vi "CameraQueryProperties.vi"(8 "error in (no error)":errorcluster, 11 "AndorSDK2 in":refnum<class "Andor3.lvclass">) -> (0 "error out":errorcluster, 1 "sensor_height":u16, 2 "sensor_width":u16, 3 "AndorSDK2 out":refnum<class "Andor3.lvclass">, 4 "cam_params":cluster{"String":string, "value":variant}[](array[cluster]) caption="params")   [LabVIEW 2010, in "Andor3.lvclass"]
uses:
  Andor3.lvclass
  Andor3.lvclass/Andor3.ctl
  <userlib>/atcoreA/atcoreA.lvlib
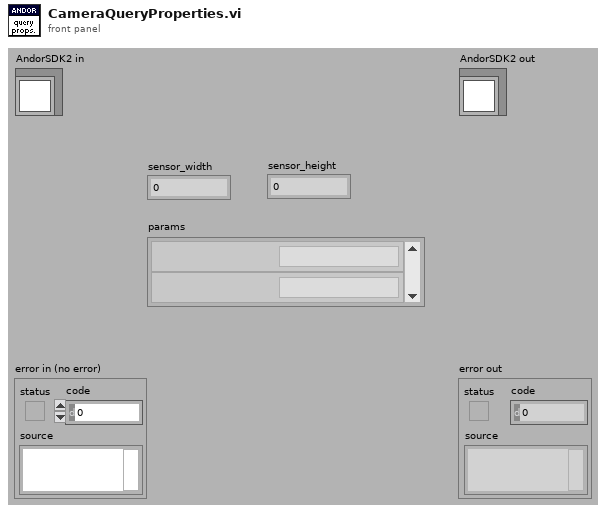
[diagram p1: front panel]
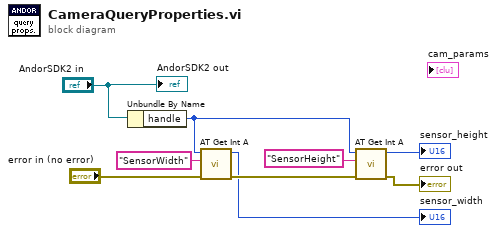
[diagram p0: block diagram]
diagram:
  n1 = Unbundle By Name("AndorSDK2 in") -> ("handle"=w1:i32)
  n2 = call <userlib>:"AT Get Int A.vi"("error in (no error)"="error in (no error)", "Feature"="SensorWidth", "Hndl"=w1) -> ("error out"=w6:errorcluster, "Value"=→"sensor_width":i64)  [unwired: 7 in]
  n3 = call <userlib>:"AT Get Int A.vi"("error in (no error)"=w6, "Feature"="SensorHeight", "Hndl"=w1) -> ("error out"=→"error out":errorcluster, "Value"=→"sensor_height":i64)  [unwired: 7 in]
  "AndorSDK2 out" <- "AndorSDK2 in"
